vi "Distort Image.vi"   [LabVIEW 2020, in "ar.lvlib" / "Image Distorter.lvclass"]
doc: "Apply distortion to the Source Image. The Destination Image will be sized to fit."
uses:
  Image Distorter.lvclass
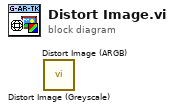
[diagram p0: block diagram]
diagram:
  n1 = call "Distort Image (Greyscale).vi"() -> ()  [unwired: 9 in, 3 out]
  n2 = call "Distort Image (ARGB).vi"() -> ()  [unwired: 9 in, 3 out]
